vi "pH Cal.vi"(0 "index":i32, 1 "pH voltage":sgl format="%.2f", 2 "Temperature":sgl format="%.2f") -> (7 "Buffers":T1(array[cluster]) {"V/T" format="%.2f"; "Buffer" format="%.2f"})   [LabVIEW 2015]
uses:
  DAQ configuration/Sensor buffer command.ctl
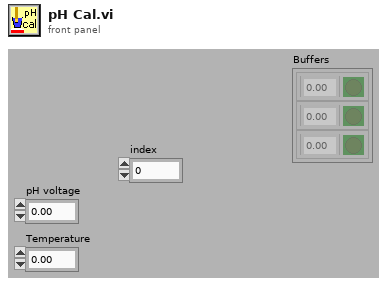
[diagram p1: front panel]
types:
  T1 = cluster{"Buffer":dbl, "Calibrated":bool, "V/T":dbl}[]
  T2 = typedef "Sensor buffer command.ctl" = enum16{"read average", "read recent", "read all", "write", "set buffer size", "Read channel config", "Write channel config", "clear"}
  T3 = enum16{"Volts", "Polynomial", "Correspondence Table", "pH", "Dissolved Oxygen"}
  T4 = typedef "Channel config.ctl" = cluster{"Channel Indices":T5[], "AI Max voltage":dbl[], "Calibration matrix":T6}
  T5 = typedef "channel identifier.ctl" = u16
  T6 = typedef "calib array.ctl" = T7[]
  T7 = typedef "conversion.ctl" = cluster{"conversion matrix":sgl[][], "units":string, "name":string, "scale type":T8, "offset (volts)":dbl, "second channel":i8, "correspondence table":T9, "offset (physical units)":dbl, "pH scale":T10, "D.O.":T11, "Photometer data":T12}
  T8 = typedef "scale type.ctl" = enum16{"Volts", "Polynomial", "Correspondence Table", "pH", "Dissolved Oxygen", "Quadratic", "Photometer"}
  T9 = typedef "correspondence table.ctl" = cluster{"physical units":dbl, "volts":dbl}[]
  T10 = typedef "pH scale.ctl" = cluster{"Buffers":cluster{"Buffer":dbl, "Calibrated":bool, "V/T":dbl}[], "Temperature":dbl}
  T11 = typedef "DO scale.ctl" = cluster{"Temperature":dbl, "K":dbl, "barometric pressure":dbl}
  T12 = typedef "Photometer calibration data.ctl" = cluster{"Dark Voltage":dbl, "Blank Voltage":dbl, "Standards":cluster{"Concentration":dbl, "Voltage":dbl}[]}
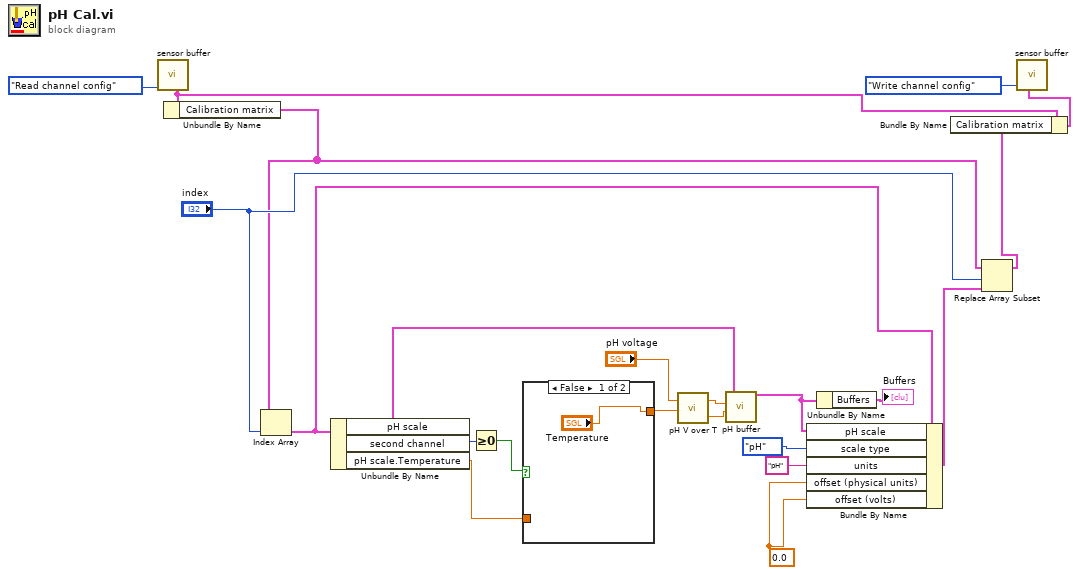
[diagram p0: block diagram]
diagram:
  w20 = 0.0 ("offset (physical units)")
  n1 = call "sensor buffer.vi"("command"=Sensor_buffer_command."Read channel config") -> ("Channel Config out"=w4:T4)  [unwired: 6 in, 4 out]
  n2 = Unbundle By Name(w4) -> ("Calibration matrix"=w5:T6)
  n3 = Index Array(array=w5, index="index") -> (element=w13:T7)
  n4 = Unbundle By Name(w13) -> ("pH scale"=w10:T10, "second channel"=w17:i8, "pH scale.Temperature"=w9:dbl)
  n5 = Greater Or Equal To 0?(x=w17) -> (x >= 0?=w18:bool)
  n6 = case shown="False" w18 {
    tunnel: ["Temperature" w24] -> w19
    tunnel: w9 -> [_ w24]
    frame False {
    }
    frame True {
    }
  }
  n7 = call "pH V over T.vi"("Temperature"=w19, "Voltage"="pH voltage") -> ("Temperature out"=w15:dbl, "V/T"=w16:dbl)
  n8 = call "pH buffer.vi"("Temperature"=w15, "V/T"=w16, "pH scale in"=w10) -> ("pH scale out"=w8:T10)  [unwired: 1 in, 1 out]
  n9 = Bundle By Name(cluster=w13, "pH scale"=w8, "scale type"=T3."pH", "units"="pH", "offset (physical units)"=w20, "offset (volts)"=w20) -> (w11:T7)
  n10 = Unbundle By Name(w8) -> ("Buffers"=→"Buffers":T1)
  n11 = Replace Array Subset(array=w5, new element=w11, index="index") -> (w1:T6)
  n12 = Bundle By Name(cluster=w4, "Calibration matrix"=w1) -> (w3:T4)
  n13 = call "sensor buffer.vi"("Channel Config"=w3, "command"=Sensor_buffer_command."Write channel config") -> ()  [unwired: 5 in, 5 out]
